vi "Read RP Calibration.vi"(8 "error in (no error)":errorcluster, 11 "RP Communicator in":refnum<class "RP Communicator.lvclass">) -> (0 "error out":errorcluster, 2 "RP Calibration":T1, 3 "RP Communicator out":refnum<class "RP Communicator.lvclass">)   [LabVIEW 2024, in "RP Communicator.lvclass"]
uses:
  RP Communicator.lvclass
  RP Communicator.lvclass/RP Communicator.ctl
  RP Channel Calibration.ctl
  RP Calibration 4ch.ctl
  RP Channel Filter.ctl
  RP Filter 4ch.ctl
  RP Calibration 2ch.ctl
  RP Calibration.ctl
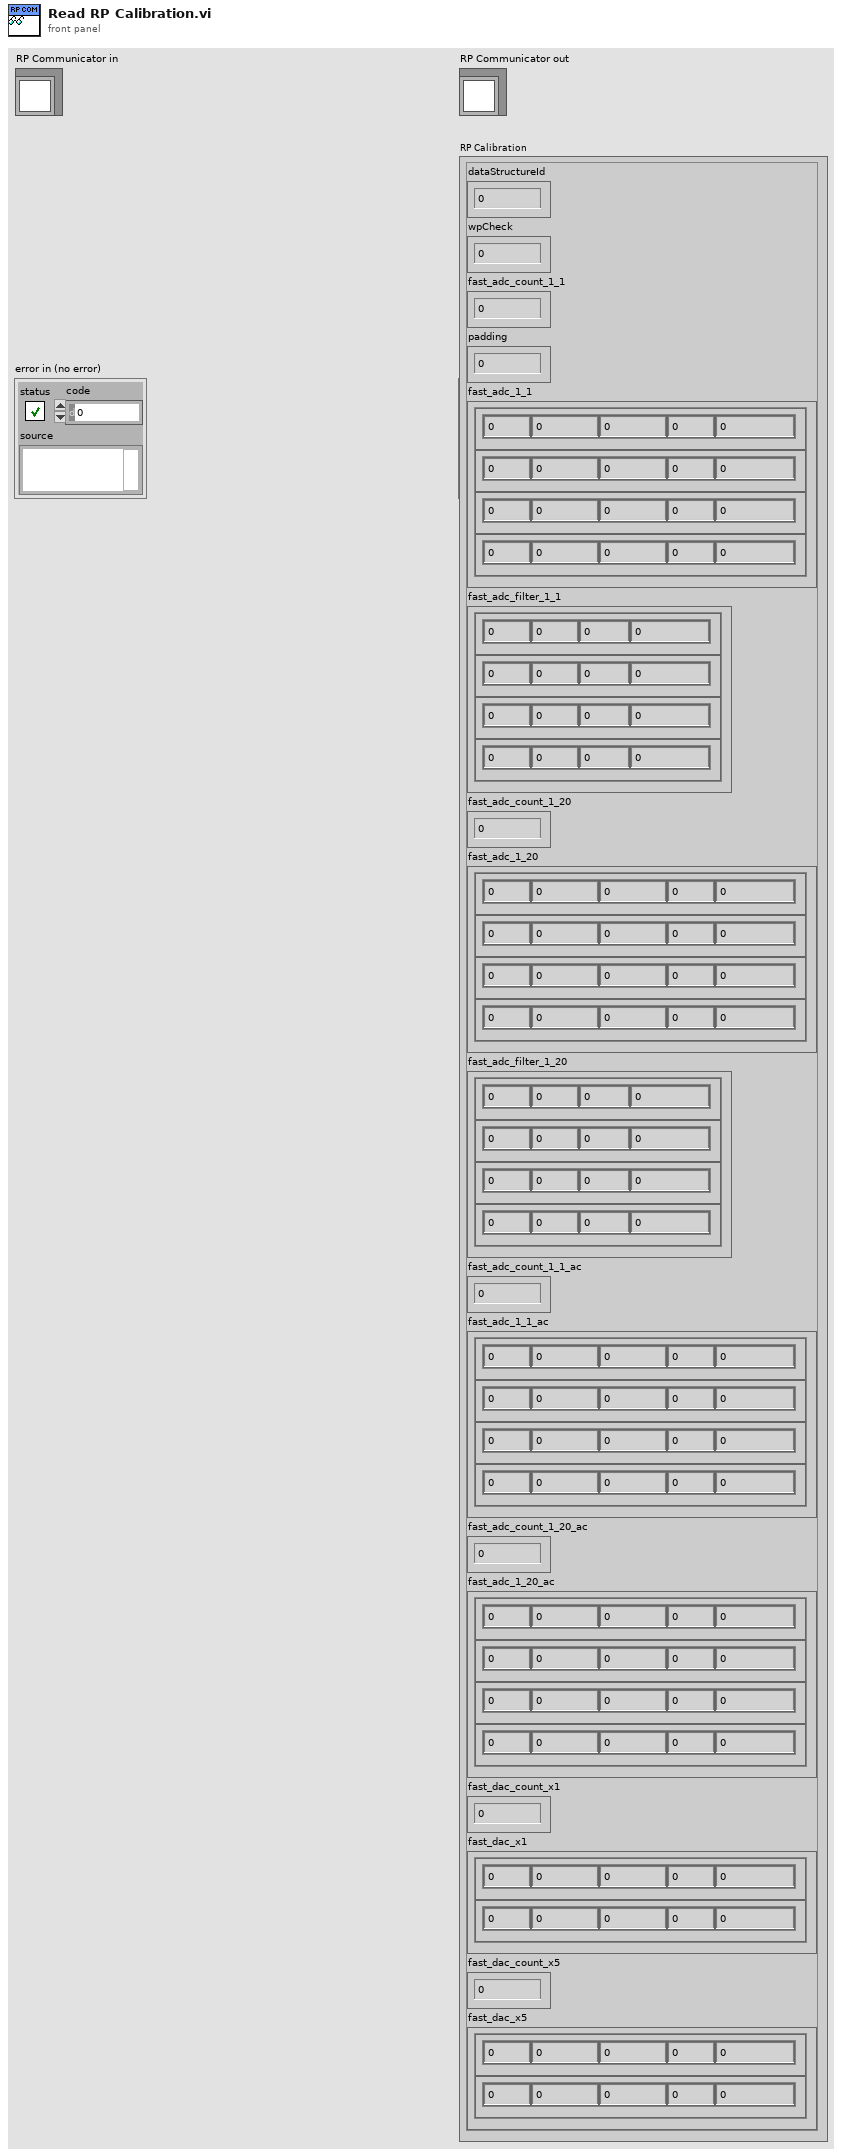
[diagram p1: front panel]
types:
  T1 = typedef "RP Calibration.ctl" = cluster{"dataStructureId":u8, "wpCheck":u8, "fast_adc_count_1_1":u16, "padding":u32, "fast_adc_1_1":T2, "fast_adc_filter_1_1":T4, "fast_adc_count_1_20":u64, "fast_adc_1_20":T2, "fast_adc_filter_1_20":T4, "fast_adc_count_1_1_ac":u64, "fast_adc_1_1_ac":T2, "fast_adc_count_1_20_ac":u64, "fast_adc_1_20_ac":T2, "fast_dac_count_x1":u64, "fast_dac_x1":T6, "fast_dac_count_x5":u64, "fast_dac_x5":T6}
  T2 = typedef "RP Calibration 4ch.ctl" = cluster{"ch_0":T3, "ch_1":T3, "ch_2":T3, "ch_3":T3}
  T3 = typedef "RP Channel Calibration.ctl" = cluster{"baseScale":sgl, "calibValue":u32, "offset":i32, "padding 2":i32, "gainCalc":dbl}
  T4 = typedef "RP Filter 4ch.ctl" = cluster{"ch_0":T5, "ch_1":T5, "ch_2":T5, "ch_3":T5}
  T5 = typedef "RP Channel Filter.ctl" = cluster{"aa":u32, "bb":u32, "pp":u32, "kk":u32}
  T6 = typedef "RP Calibration 2ch.ctl" = cluster{"ch_0":T3, "ch_1":T3}
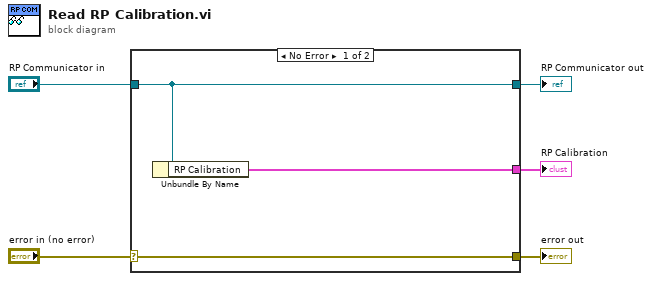
[diagram p0: block diagram]
diagram:
  n1 = case shown="No Error" "error in (no error)" {
    selector: "error in (no error)" -> [w8 w9]
    tunnel: [w8 w9] -> w4
    tunnel: [w7 w10] -> w2
    tunnel: "RP Communicator in" -> [w7 w10]
    tunnel: [w6 _] -> w1
    frame No Error {
      n2 = Unbundle By Name(w7) -> ("RP Calibration"=w6:T1)
    }
    frame Error {
    }
  }
  "error out" <- w4
  "RP Communicator out" <- w2
  "RP Calibration" <- w1
